vi "SpecAnState.vi"(7 "Set Boolean":bool, 11 "State In":string) -> (3 "State Out":string)   [LabVIEW 2014, in "SpecAnModule.lvlib"]
uses:
  SpecAnModule.lvlib
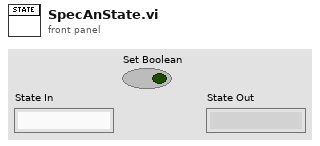
[diagram p1: front panel]
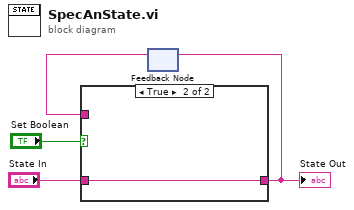
[diagram p0: block diagram]
diagram:
  n1 = feedback #1() -> (w1:string)  [unwired: 1 in]
  n2 = case shown="True" "Set Boolean" {
    tunnel: "State In" -> [_ w6]
    tunnel: [w5 w6] -> w2
    tunnel: w1 -> [w5 _]
    frame False {
    }
    frame True {
    }
  }
  "State Out" <- w2
  n3 = feedback-in #1(w2) -> ()
